vi "Parse Parameters File.vi"(8 "error in":errorcluster, 11 "path to XML document":path caption="path to parameters xml") -> (0 "error out":errorcluster, 1 "ports":T1[](array[typedef]), 3 "path to XML document out":path caption="path to parameters xml")   [LabVIEW 2020, in "ARINC 429 Import.lvlib"]
uses:
  ARINC 429 Import.lvlib
  Shared/VS Channels Definition for All Labels on Hardware Channel.ctl
  Shared/Direction.ctl
  Shared/VS Channels Definition for Label.ctl
  Shared/VS Channel Definition for Parameter.ctl
  Shared/Parameter Definition.ctl
  <vilib>/NI/NI VeriStand Encoding and Decoding/Encoding.ctl
  Shared/Transfer Type.ctl
  <vilib>/xml/Load XML File.vi
  Read Tag Element (U16).vi
  Read Tag Element (Direction).vi
  <vilib>/xml/NI_XML.lvlib
  <resource>/objmgr/DOMUserDefRef.rc
  <vilib>/NI/NI VeriStand Encoding and Decoding/Encoding and Decoding.lvlib
panel:
  out "parse errors":string
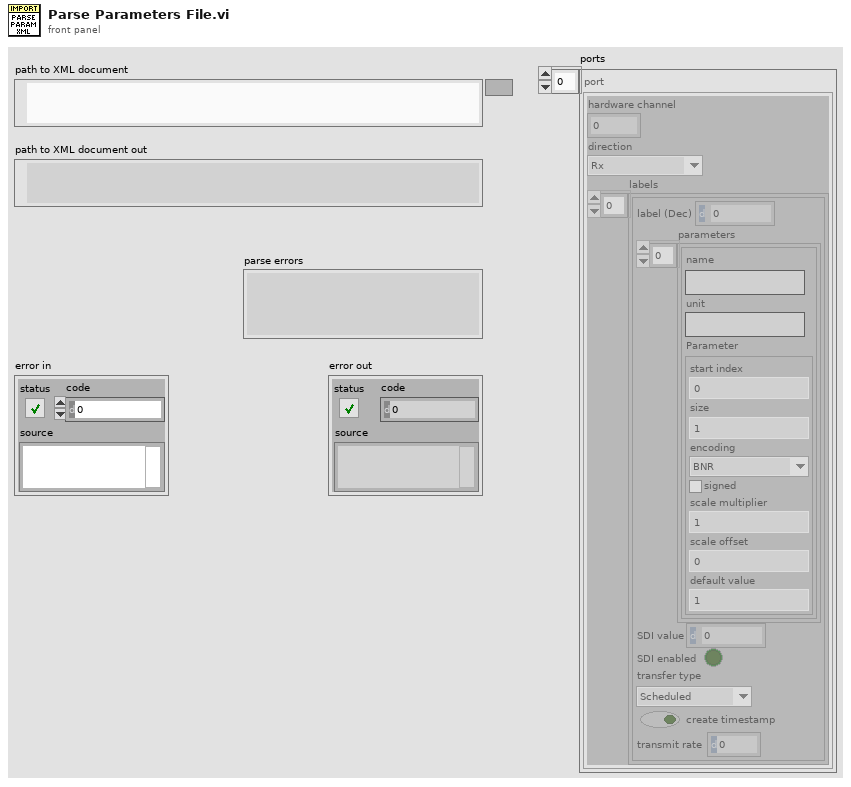
[diagram p1: front panel]
types:
  T1 = typedef "VS Channels Definition for All Labels on Hardware Channel.ctl" = cluster{"hardware channel":i32, "direction":T2, "labels":T3[]}
  T2 = typedef "Direction.ctl" = enum16{"Rx", "Tx"}
  T3 = typedef "VS Channels Definition for Label.ctl" = cluster{"label (Dec)":u32, "parameters":T4[], "SDI value":u8, "SDI enabled":bool, "transfer type":T7, "create timestamp":bool, "transmit rate":u32}
  T4 = typedef "VS Channel Definition for Parameter.ctl" = cluster{"name":string, "unit":string, "Parameter":T5}
  T5 = typedef "Parameter Definition.ctl" = cluster{"start index":i32, "size":i32, "encoding":T6, "signed":bool, "scale multiplier":dbl, "scale offset":dbl, "default value":dbl}
  T6 = typedef "Encoding and Decoding.lvlib/Encoding.ctl" = enum16{"BNR", "BCD", "Discrete"}
  T7 = typedef "Transfer Type.ctl" = enum16{"Scheduled", "Acyclic", "Block", "Strobe"}
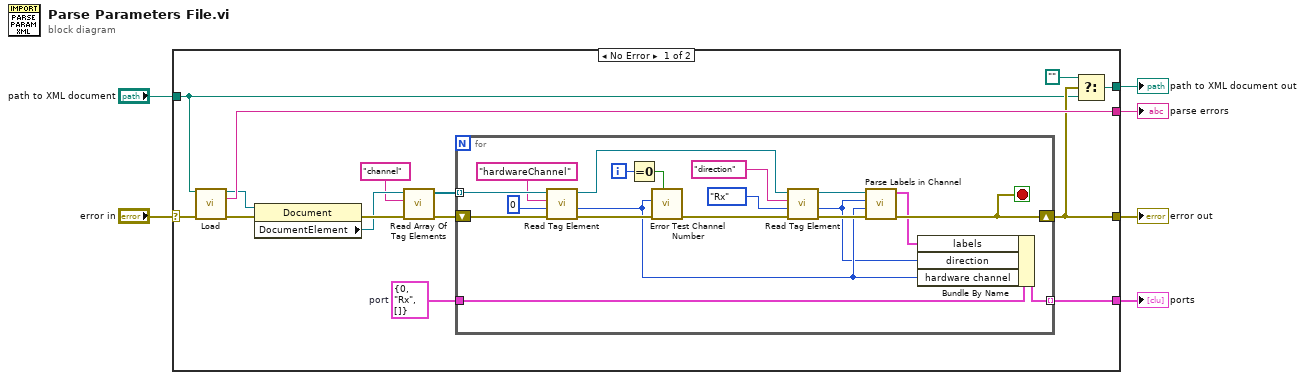
[diagram p0: block diagram]
diagram:
  n1 = case shown="No Error" "error in" {
    selector: "error in" -> [w12 w41]
    tunnel: [w21 _] -> w6
    tunnel: [w19 _] -> w5
    tunnel: [w11 w41] -> w4
    tunnel: "path to XML document" -> [w9 _]
    tunnel: [w10 _] -> w1
    frame No Error {
      w7 = T1 {"hardware channel"=0, "direction"=enum."Rx", "labels"=[]}  # port
      n2 = call-poly <vilib>:"Load.vi"("path to XML document"=w9, "error in (no error)"=w12) -> ("DOM document out"=w20:refnum<k20>, "parse errors"=w21:string, "error out"=w18:errorcluster)  [unwired: 11 in]
      n3 = property class="Document"(reference=w20, error in=w18) -> (error out=w16:errorcluster, "DocumentElement"=w15:refnum<k20>)  [unwired: 1 out]
      n4 = call "Read Array Of Tag Elements.vi"("error in"=w16, "tag name"="channel" ("Tag Name"), "node in"=w15) -> ("error out"=w17:errorcluster, "array of elements"=w14:refnum<k20>[])  [unwired: 7 in]
      n5 = for {
        tunnel: w14 -> [w40] mode=indexing
        shift-right: [w29] -> w11
        shift-left: w17 -> [w36]
        tunnel: [w39] -> w19 mode=indexing
        tunnel: w7 -> [w22]
        i -> [w25]
        stop <- w29 stop-if-true
        n6 = call-poly "Read Tag Element.vi"("error in"=w36, "default"=u16 0, "Tag Name"="hardwareChannel", "node in"=w40) -> ("error out"=w33:errorcluster, "value"=w26:u16, "node out"=w38:refnum<k20>)  [unwired: 5 in]
        n7 = Equal To 0?(x=w25) -> (x = 0?=w24:bool)
        n8 = call "Error Test Channel Number.vi"("reset (F)"=w24, "error in"=w33, "channel #"=w26) -> ("error out"=w32:errorcluster)  [unwired: 8 in]
        n9 = call-poly "Read Tag Element.vi"("error in"=w32, "default"=Direction."Rx", "Tag Name"="direction", "node in"=w38) -> ("error out"=w31:errorcluster, "value"=w23:T2, "node out"=w30:refnum<k20>)  [unwired: 5 in]
        n10 = call "Parse Labels in Channel.vi"("error in"=w31, "channel #"=w26, "direction"=w23, "node in"=w30) -> ("error out"=w29:errorcluster, "labels"=w28:T3[])  [unwired: 6 in]
        n11 = Bundle By Name(cluster=w22, "labels"=w28, "direction"=w23, "hardware channel"=w26) -> (w39:T1)
      }
      n12 = Select(t=path "", s=w11, f=w9) -> (s? t:f=w10:path)
    }
    frame Error {
    }
  }
  "parse errors" <- w6
  "ports" <- w5
  "error out" <- w4
  "path to XML document out" <- w1
